vi "步响应V0V1.vi"(3 "步响应计算参数 in":T1, 4 "NbOfPointsToAverage":dbl=1000.0, 5 "行程 in":dbl[](array[numeric])) -> (0 "步响应计算参数 out":T1, 2 "行程 out":dbl[](array[numeric]))   [LabVIEW 2013]
panel:
  out "SEN":string
  out "SEN":dbl
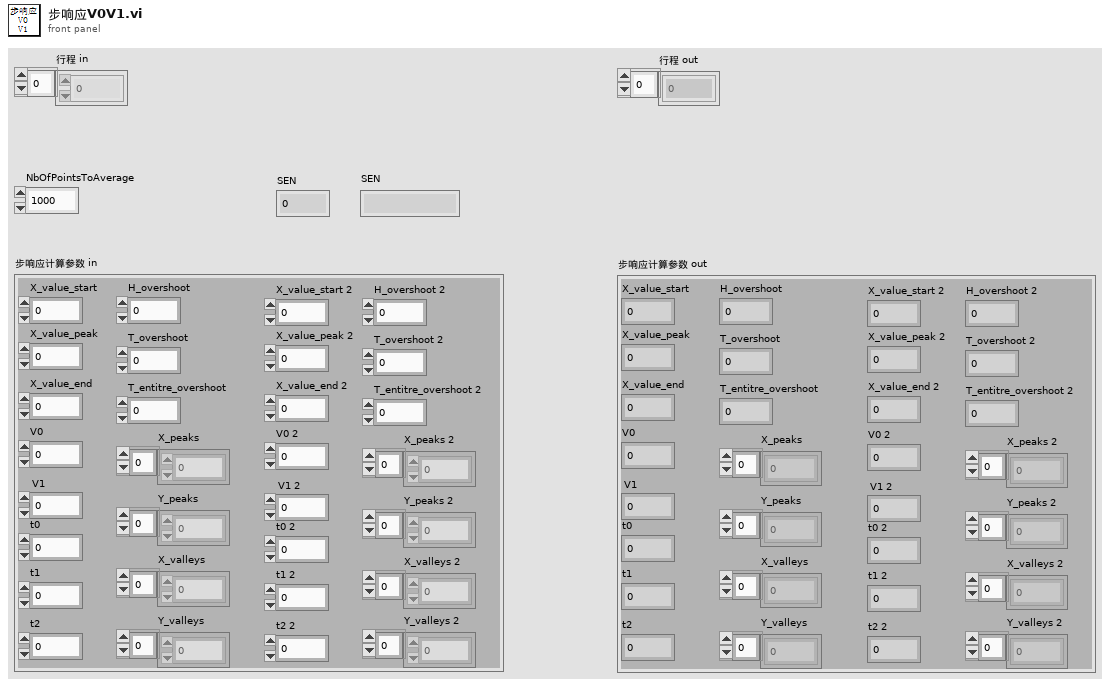
[diagram p1: front panel]
types:
  T1 = cluster{"X_value_start":dbl, "X_value_peak":dbl, "t1":dbl, "X_value_end":dbl, "V0":dbl, "V1":dbl, "t0":dbl, "X_peaks":dbl[], "X_valleys":dbl[], "Y_peaks":dbl[], "Y_valleys":dbl[], "t2":dbl, "H_overshoot":dbl, "T_overshoot":dbl, "T_entitre_overshoot":dbl, "X_value_start 2":dbl, "X_value_peak 2":dbl, "t1 2":dbl, "X_value_end 2":dbl, "V0 2":dbl, "V1 2":dbl, "t0 2":dbl, "X_peaks 2":dbl[], "X_valleys 2":dbl[], "Y_peaks 2":dbl[], "t2 2":dbl, "H_overshoot 2":dbl, "T_overshoot 2":dbl, "T_entitre_overshoot 2":dbl, "Y_valleys 2":dbl[]}
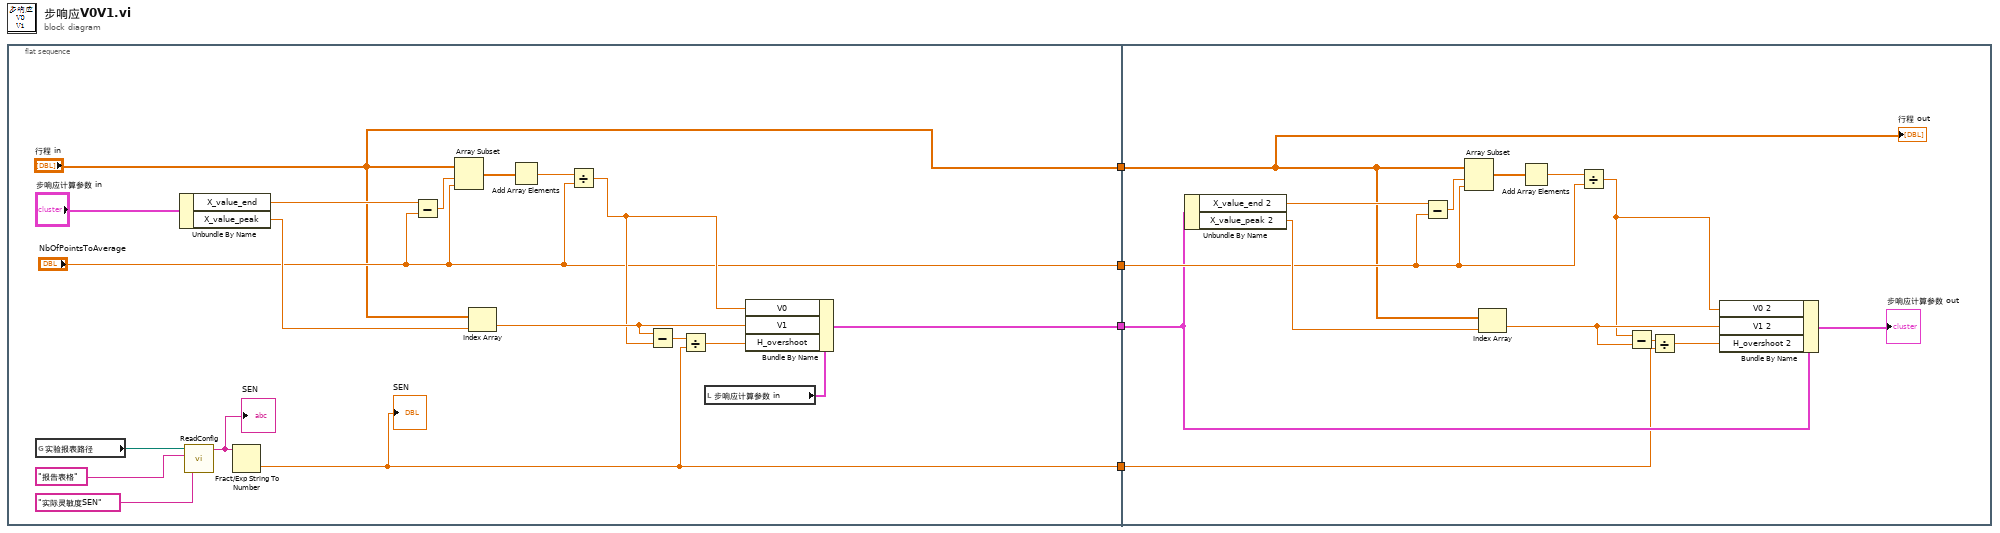
[diagram p0: block diagram]
diagram:
  n1 = flat-sequence {
    tunnel: ["NbOfPointsToAverage"] -> w4
    tunnel: ["行程 in"] -> w3
    tunnel: [w12] -> w2
    tunnel: [w5] -> w1
    tunnel: w4 -> [w29]
    tunnel: w3 -> [w28]
    tunnel: w2 -> [w27]
    tunnel: w1 -> [w24]
    frame #0 {
      n2 = global read "实验报表路径.vi" "实验报表路径"() -> (w9:path)
      n3 = Unbundle By Name("步响应计算参数 in") -> ("X_value_end"=w20:dbl, "X_value_peak"=w19:dbl)
      n4 = call "ReadConfig.vi"("Key"="实际灵敏度SEN", "Section"="报告表格", "Path"=w9) -> ("Value"=w6:string)  [unwired: 1 in, 2 out]
      "SEN" <- w6
      n5 = Fract/Exp String To Number(string=w6) -> (number=w5:dbl)  [unwired: 3 in, 1 out]
      "SEN" <- w5
      n6 = Subtract(x=w20, y="NbOfPointsToAverage") -> (x-y=w21:dbl)
      n7 = Array Subset(array="行程 in", index=w21, length="NbOfPointsToAverage") -> (w23:dbl[])
      n8 = Index Array(array="行程 in", index=w19) -> (element=w18:dbl)
      n9 = Add Array Elements(numeric array=w23) -> (sum=w22:dbl)
      n10 = Divide(x=w22, y="NbOfPointsToAverage") -> (x/y=w17:dbl)
      n11 = Subtract(x=w18, y=w17) -> (x-y=w8:dbl)
      n12 = Divide(x=w8, y=w5) -> (x/y=w7:dbl)
      n13 = local read "步响应计算参数 in"() -> (w15:T1)
      n14 = Bundle By Name(cluster=w15, "V0"=w17, "V1"=w18, "H_overshoot"=w7) -> (w12:T1)
    }
    frame #1 {
      n15 = Unbundle By Name(w27) -> ("X_value_end 2"=w33:dbl, "X_value_peak 2"=w34:dbl)
      n16 = Subtract(x=w33, y=w29) -> (x-y=w32:dbl)
      n17 = Array Subset(array=w28, index=w32, length=w29) -> (w30:dbl[])
      n18 = Index Array(array=w28, index=w34) -> (element=w36:dbl)
      n19 = Add Array Elements(numeric array=w30) -> (sum=w31:dbl)
      n20 = Divide(x=w31, y=w29) -> (x/y=w35:dbl)
      n21 = Subtract(x=w35, y=w36) -> (x-y=w26:dbl)
      n22 = Divide(x=w26, y=w24) -> (x/y=w25:dbl)
      n23 = Bundle By Name(cluster=w27, "V0 2"=w35, "V1 2"=w36, "H_overshoot 2"=w25) -> (→"步响应计算参数 out":T1)
      "行程 out" <- w28
    }
  }
